vi "SLSC Populate Module Tree.vi"(8 "error in (no error)":errorcluster, 11 "Device Item Ref in":T8 format="%.0x") -> (0 "error out":errorcluster, 1 "SLSC Module Name":string, 2 "SLSC EDS module":T1, 3 "Device Item Ref out":T8 format="%.0x", 4 "Initialized?":bool)   [LabVIEW 2020, in "SLSC EDS System Explorer.lvlib"]
uses:
  System Explorer/SLSC EDS System Explorer.lvlib
  <vilib>/NI VeriStand/Custom Device API/Custom Device Item Ref.ctl
  SLSC EDS API/JSON parsing/EDSjsonStructure.ctl
  SLSC EDS API/JSON parsing/enum.ctl
  SLSC EDS API/JSON parsing/property.ctl
  SLSC EDS API/JSON parsing/command.ctl
  SLSC EDS API/JSON parsing/scale.ctl
  SLSC EDS API/JSON parsing/physicalChannel.ctl
  SLSC EDS API/JSON parsing/register.ctl
  Shared/Constants.vi
  <vilib>/NI VeriStand/Custom Device API/Get Item Property (U32).vi
  <vilib>/NI VeriStand/Custom Device API/Custom Device API.lvlib
  Shared/SLSC EDS Shared.lvlib
  SLSC CD System Explorer.lvlib
panel:
  # "not working\nregisterMap->registers->initialValue"
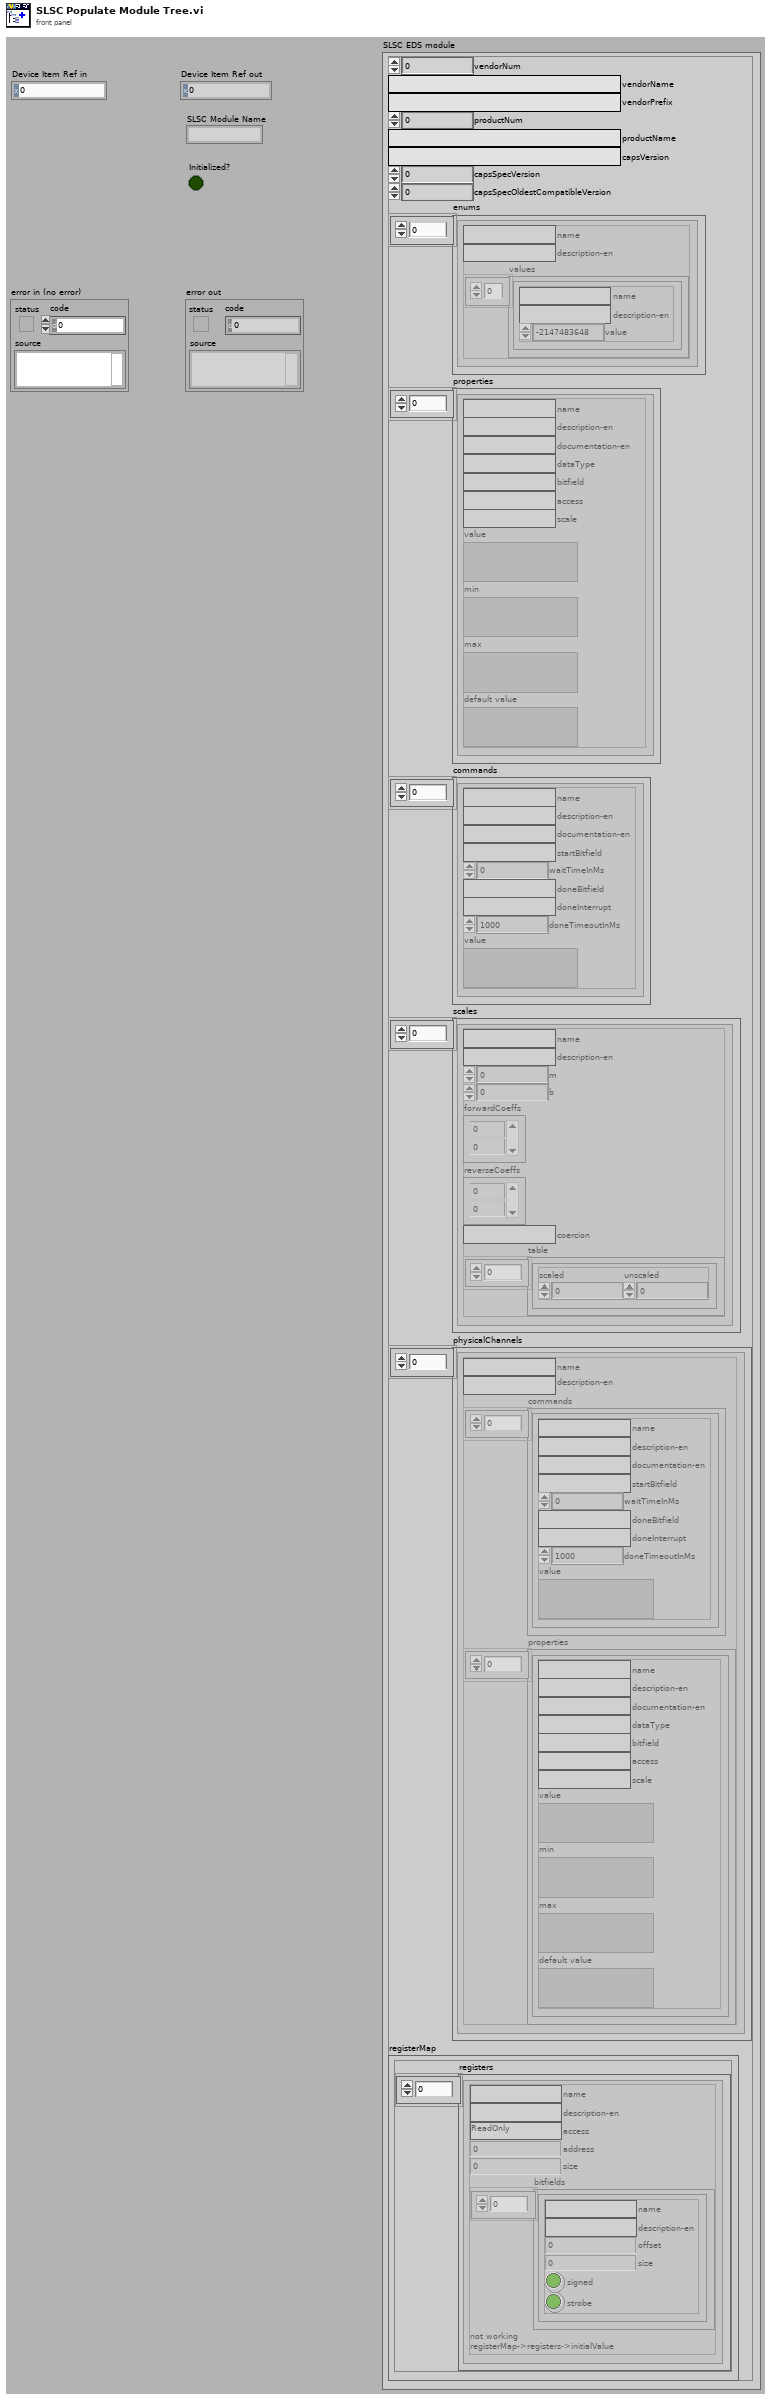
[diagram p1: front panel]
types:
  T1 = typedef "EDSjsonStructure.ctl" = cluster{"vendorNum":u32, "vendorName":string, "vendorPrefix":string, "productNum":u32, "productName":string, "capsVersion":string, "capsSpecVersion":u32, "capsSpecOldestCompatibleVersion":u32, "enums":T2[], "properties":T3[], "commands":T4[], "scales":T5[], "physicalChannels":T6[], "registerMap":cluster{"registers":T7[]}}
  T2 = typedef "enum.ctl" = cluster{"name":string, "description-en":string, "values":cluster{"name":string, "description-en":string, "value":i32}[]}
  T3 = typedef "property.ctl" = cluster{"name":string, "description-en":string, "documentation-en":string, "dataType":string, "bitfield":string, "access":string, "scale":string, "value":variant, "min":variant, "max":variant, "default value":variant}
  T4 = typedef "command.ctl" = cluster{"name":string, "description-en":string, "documentation-en":string, "startBitfield":string, "waitTimeInMs":i32, "doneBitfield":string, "doneInterrupt":string, "doneTimeoutInMs":i32, "value":variant}
  T5 = typedef "scale.ctl" = cluster{"name":string, "description-en":string, "m":dbl, "b":dbl, "forwardCoeffs":dbl[], "reverseCoeffs":dbl[], "coercion":string, "table":cluster{"scaled":dbl, "unscaled":dbl}[]}
  T6 = typedef "physicalChannel.ctl" = cluster{"name":string, "description-en":string, "commands":T4[], "properties":T3[]}
  T7 = typedef "register.ctl" = cluster{"name":string, "description-en":string, "access":string, "address":u32, "size":u32, "bitfields":cluster{"name":string, "description-en":string, "offset":u32, "size":u32, "signed":bool, "strobe":bool}[]}
  T8 = typedef "Custom Device API.lvlib/Custom Device Item Ref.ctl" = u64
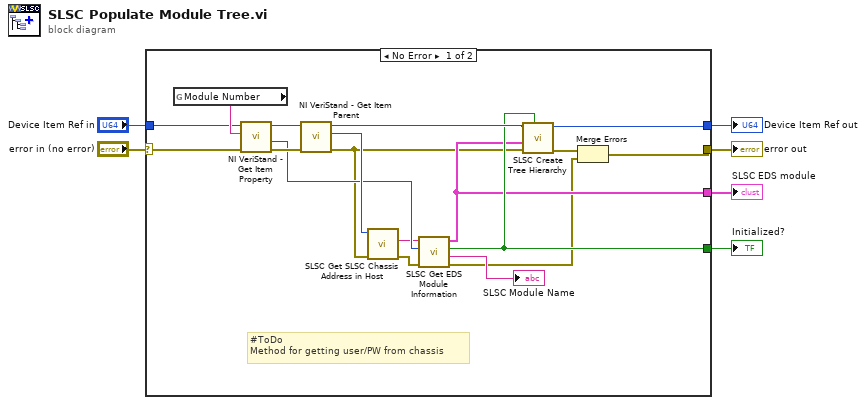
[diagram p0: block diagram]
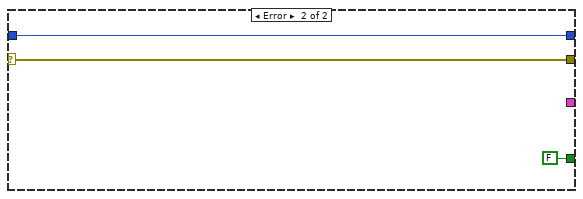
[diagram p2: hidden frame]
diagram:
  n1 = case shown="No Error" "error in (no error)" {
    selector: "error in (no error)" -> [w12 w27]
    tunnel: [w8 w27] -> w6
    tunnel: [w15 w26] -> w4
    tunnel: "Device Item Ref in" -> [w11 w26]
    tunnel: [w13 FALSE ("Initialized?")] -> w2
    tunnel: [w10 _] -> w1
    frame No Error {
      # "#ToDo\nMethod for getting user/PW from chassis"
      n2 = global read "Constants.vi" "Module Number"() -> (w24:string)
      n3 = call-poly <vilib>:"NI VeriStand - Get Item Property.vi"("error in (no error)"=w12, "Property Name"=w24, "Item Ref in"=w11) -> ("error out"=w21:errorcluster, "Value"=w19:u32, "Item Ref out"=w22:T8)  [unwired: 5 in, 1 out]
      n4 = call <vilib>:"NI VeriStand - Get Item Parent.vi"("error in (no error)"=w21, "Item Ref in"=w22) -> ("error out"=w9:errorcluster, "Parent Ref"=w23:T8, "Item Ref out"=w16:T8)  [unwired: 6 in, 1 out]
      n5 = call "SLSC Get SLSC Chassis Address in Host.vi"("error in (no error)"=w9, "Parent Ref"=w23) -> ("error out"=w20:errorcluster, "IP Address"=w18:string)  [unwired: 6 in, 2 out]
      n6 = call "SLSC Get EDS Module Information.vi"("error in (no error)"=w20, "Slot #"=w19, "Chassis IP Address"=w18) -> ("error out"=w7:errorcluster, "SLSC Module Name"=→"SLSC Module Name":string, "Initialized?"=w13:bool, "SLSC EDS module"=w10:T1)  [unwired: 5 in]
      n7 = call "SLSC Create Tree Hierarchy.vi"("Initialized?"=w13, "error in (no error)"=w9, "SLSC EDS module"=w10, "Item Ref in"=w16) -> ("error out"=w14:errorcluster, "Parent Ref out"=w15:T8)  [unwired: 6 in]
      n8 = Merge Errors(w14, w7) -> (w8:errorcluster)
    }
    frame Error {
    }
  }
  "error out" <- w6
  "Device Item Ref out" <- w4
  "Initialized?" <- w2
  "SLSC EDS module" <- w1
